vi "pidENC.vi"(1 "当前值":dbl, 2 "目标值":dbl, 3 "kd":dbl, 4 "ki":dbl, 5 "kp":dbl) -> (0 "输出":dbl)   [LabVIEW 2022 SP3]
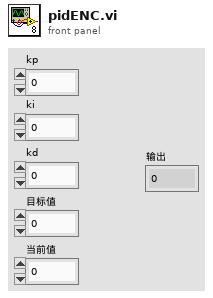
[diagram p1: front panel]
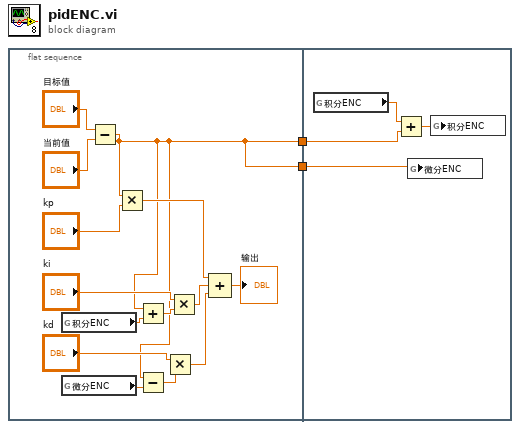
[diagram p0: block diagram]
diagram:
  n1 = flat-sequence {
    tunnel: [w3] -> w2
    tunnel: [w3] -> w1
    tunnel: w2 -> [w18]
    tunnel: w1 -> [w17]
    frame #0 {
      n2 = global read "全局变量.vi" "积分ENC"() -> (w6:dbl)
      n3 = global read "全局变量.vi" "微分ENC"() -> (w4:dbl)
      n4 = Subtract(x="目标值", y="当前值") -> (x-y=w3:dbl)
      n5 = Multiply(x=w3, y="kp") -> (x*y=w13:dbl)
      n6 = Add(x=w3, y=w6) -> (x+y=w7:dbl)
      n7 = Subtract(x=w3, y=w4) -> (x-y=w5:dbl)
      n8 = Multiply(x="kd", y=w5) -> (x*y=w11:dbl)
      n9 = Multiply(x="ki", y=w7) -> (x*y=w9:dbl)
      n10 = Compound Arithmetic op=ADD(w13, w9, w11) -> (→"输出":dbl)
    }
    frame #1 {
      n11 = global read "全局变量.vi" "积分ENC"() -> (w19:dbl)
      n12 = Add(x=w19, y=w18) -> (x+y=w20:dbl)
      n13 = global write "全局变量.vi" "微分ENC"(w17) -> ()
      n14 = global write "全局变量.vi" "积分ENC"(w20) -> ()
    }
  }
